vi "Queue Global.vi"(7 "Set?":bool, 10 "Queue in":refnum<class "Message Enqueuer.lvclass">) -> (2 "Queue out":refnum<class "Message Enqueuer.lvclass">)   [LabVIEW 2018, in "Monitored Actor.lvlib" / "Actor Monitor.lvclass"]
doc: "Functional global to store the Actor Monitor's Queue\n\nCopyright: MGI\nAuthored by: Derek Trepanier"
uses:
  Actor Monitor.lvclass
  <vilib>/ActorFramework/Message Enqueuer/Message Enqueuer.lvclass
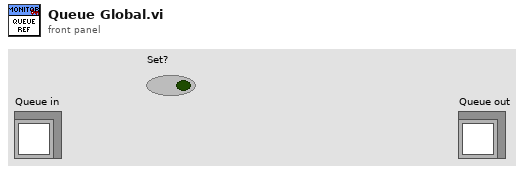
[diagram p1: front panel]
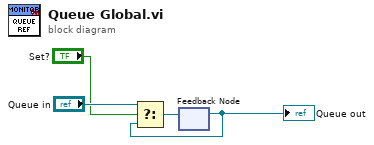
[diagram p0: block diagram]
diagram:
  n1 = feedback #1() -> (w2:refnum<class "Message Enqueuer.lvclass">)  [unwired: 1 in]
  "Queue out" <- w2
  n2 = Select(t="Queue in", s="Set?", f=w2) -> (s? t:f=w3:refnum<class "Message Enqueuer.lvclass">)
  n3 = feedback-in #1(w3) -> ()
